vi "Test.vi"() -> ()   [LabVIEW 2020]
uses:
  Supporting Files/Axis Parameters.ctl
panel:
  out "While Loop":string
  in  "stop":bool
  in  "Path":string
  out "output cluster":T1 {"VPSPEED" format="%#_4g"; "AXISSTATUS" format="%#_4g"; "FE" format="%#_4g"; "MPOS" format="%#_4g"; "NTYPE" format="%#_4g"; "MTYPE" format="%#_4g"; "RS_LIMIT" format="%#_4g"; "FS_LIMIT" format="%#_4g"; "FH_IN" format="%#_4g"; "DATUM_IN" format="%#_4g"; "REV_IN" format="%#_4g"; "FWD_IN" format="%#_4g"; "REP_DIST" format="%#_4g"; "SERVO" format="%#_4g"; "DAC" format="%#_4g"; "FE_LIMIT" format="%#_4g"; "JOGSPEED" format="%#_4g"; "CREEP" format="%#_4g"; "DECEL" format="%#_4g"; "ACCEL" format="%#_4g"; "SPEED" format="%#_4g"; "UNITS" format="%#_4g"; "VFF_GAIN" format="%#_4g"; "0V_GAIN" format="%#_4g"; "D_GAIN" format="%#_4g"; "I_GAIN" format="%#_4g"; "P_GAIN" format="%#_4g"; "ATYPE" format="%#_4g"}
  in  "error in (no error)":errorcluster
  out "error out":errorcluster
  out "Axis Parameter Values":string[][](table)
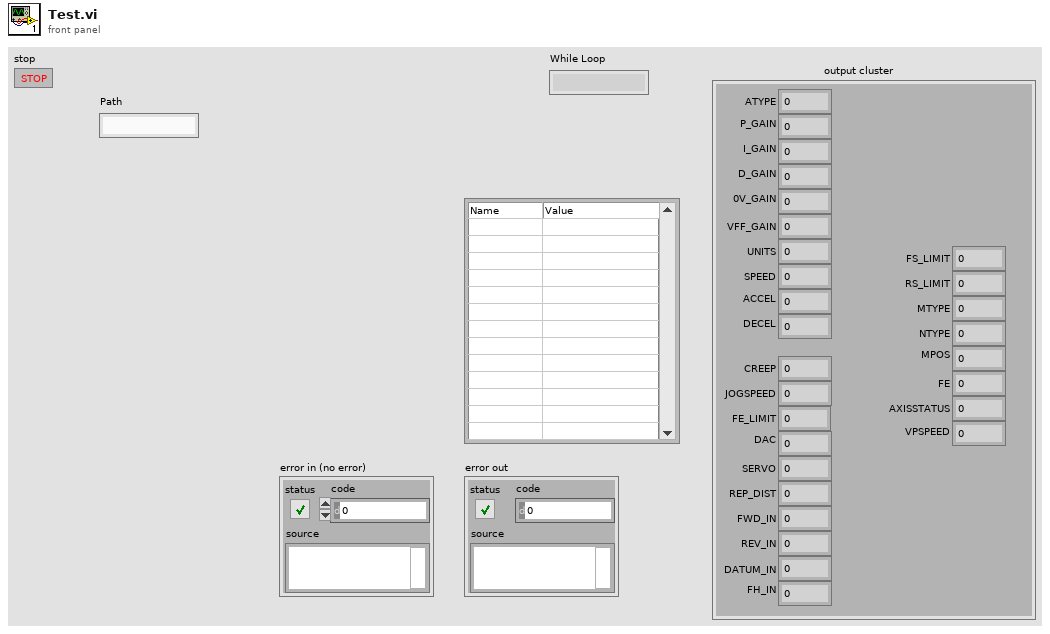
[diagram p1: front panel]
types:
  T1 = typedef "Axis Parameters.ctl" = cluster{"ATYPE":dbl, "P_GAIN":dbl, "I_GAIN":dbl, "D_GAIN":dbl, "0V_GAIN":dbl, "VFF_GAIN":dbl, "UNITS":dbl, "SPEED":dbl, "ACCEL":dbl, "DECEL":dbl, "CREEP":dbl, "JOGSPEED":dbl, "FE_LIMIT":dbl, "DAC":dbl, "SERVO":dbl, "REP_DIST":dbl, "FWD_IN":dbl, "REV_IN":dbl, "DATUM_IN":dbl, "FH_IN":dbl, "FS_LIMIT":dbl, "RS_LIMIT":dbl, "MTYPE":dbl, "NTYPE":dbl, "MPOS":dbl, "FE":dbl, "AXISSTATUS":dbl, "VPSPEED":dbl}
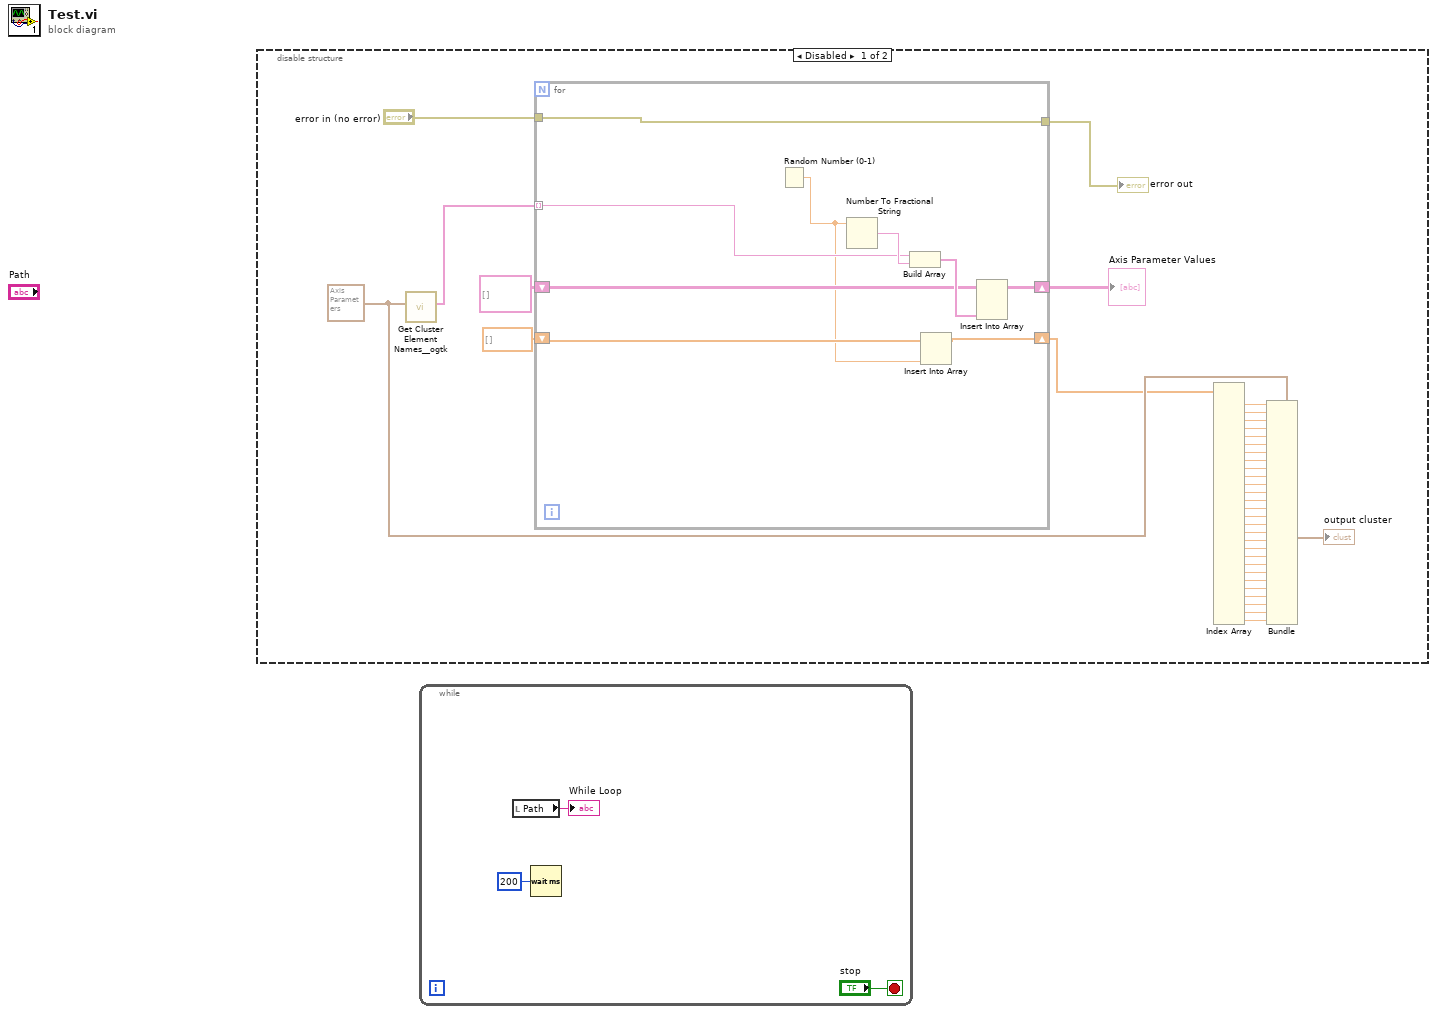
[diagram p0: block diagram]
diagram:
  n1 = disable-structure shown="Disabled" {
    frame Disabled {
      w31 = T1 {"ATYPE"=0.0, "P_GAIN"=0.0, "I_GAIN"=0.0, "D_GAIN"=0.0, "0V_GAIN"=0.0, "VFF_GAIN"=0.0, "UNITS"=0.0, "SPEED"=0.0, "ACCEL"=0.0, "DECEL"=0.0, "CREEP"=0.0, "JOGSPEED"=0.0, "FE_LIMIT"=0.0, "DAC"=0.0, "SERVO"=0.0, "REP_DIST"=0.0, "FWD_IN"=0.0, "REV_IN"=0.0, "DATUM_IN"=0.0, "FH_IN"=0.0, "FS_LIMIT"=0.0, "RS_LIMIT"=0.0, "MTYPE"=0.0, "NTYPE"=0.0, "MPOS"=0.0, "FE"=0.0, "AXISSTATUS"=0.0, "VPSPEED"=0.0}
      n2 = call <userlib>:"Get Cluster Element Names__ogtk.vi"("Cluster"=w31) -> ("Element Names"=w32:string[])  [unwired: 9 in, 1 out]
      n3 = for {
        tunnel: w32 -> [w39] mode=indexing
        tunnel: "error in (no error)" -> [w40]
        shift-right: [w44] -> w34
        shift-left: string[][] [] ("Axis Parameters") -> [w45]
        tunnel: [w40] -> w37
        shift-right: [w42] -> w30
        shift-left: dbl[] [] ("Axis Parameters") -> [w41]
        n4 = Random Number (0-1)() -> (number: 0 to 1=w38:dbl)
        n5 = Number To Fractional String(number=w38) -> (F-format string=w43:string)  [unwired: 3 in]
        n6 = Build Array(w39, w43) -> (w46:string[])
        n7 = Insert Into Array(array=w41, new element=w38) -> (w42:dbl[])  [unwired: 1 in]
        n8 = Insert Into Array(array=w45, new element=w46) -> (w44:string[][])  [unwired: 2 in]
      }
      "Axis Parameter Values" <- w34
      "error out" <- w37
      n9 = Index Array(array=w30) -> (element #1=w29:dbl, element #2=w27:dbl, element #3=w26:dbl, element #4=w25:dbl, element #5=w24:dbl, element #6=w23:dbl, element #7=w22:dbl, element #8=w21:dbl, element #9=w20:dbl, element #10=w19:dbl, element #11=w18:dbl, element #12=w17:dbl, element #13=w16:dbl, element #14=w15:dbl, element #15=w14:dbl, element #16=w13:dbl, element #17=w12:dbl, element #18=w11:dbl, element #19=w10:dbl, element #20=w9:dbl, element #21=w8:dbl, element #22=w7:dbl, element #23=w6:dbl, element #24=w5:dbl, element #25=w4:dbl, element #26=w3:dbl, element #27=w2:dbl, element #28=w1:dbl)  [unwired: 28 in]
      n10 = Bundle(cluster=w31, "ATYPE"=w29, "P_GAIN"=w27, "I_GAIN"=w26, "D_GAIN"=w25, "0V_GAIN"=w24, "VFF_GAIN"=w23, "UNITS"=w22, "SPEED"=w21, "ACCEL"=w20, "DECEL"=w19, "CREEP"=w18, "JOGSPEED"=w17, "FE_LIMIT"=w16, "DAC"=w15, "SERVO"=w14, "REP_DIST"=w13, "FWD_IN"=w12, "REV_IN"=w11, "DATUM_IN"=w10, "FH_IN"=w9, "FS_LIMIT"=w8, "RS_LIMIT"=w7, "MTYPE"=w6, "NTYPE"=w5, "MPOS"=w4, "FE"=w3, "AXISSTATUS"=w2, "VPSPEED"=w1) -> (→"output cluster":T1)
    }
    frame Enabled {
    }
  }
  n11 = while {
    stop <- "stop" stop-if-true
    n12 = local read "Path"() -> (→"While Loop":string)
    n13 = Wait (ms)(milliseconds to wait=u32 200) -> ()  [unwired: 1 out]
  }
